vi "Format Error Properties.vi"(8 "error in (no error)":errorcluster, 11 "CtrlTerm Ref":refnum<vi>) -> (0 "error out":errorcluster, 2 "Changed?":bool)   [LabVIEW 2020]
uses:
  <vilib>/Utility/miscctls.llb/LVSelectionTypeDef.ctl
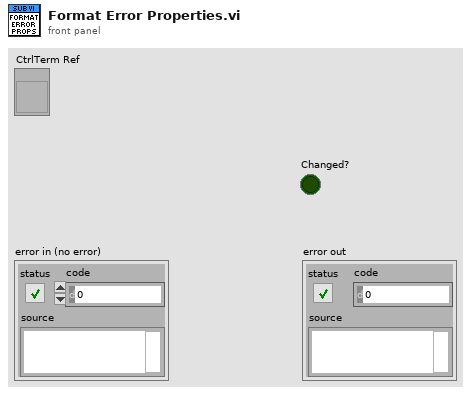
[diagram p1: front panel]
types:
  T1 = typedef "LVSelectionTypeDef.ctl" = cluster{"Selection Start":u32, "Selection End":u32}
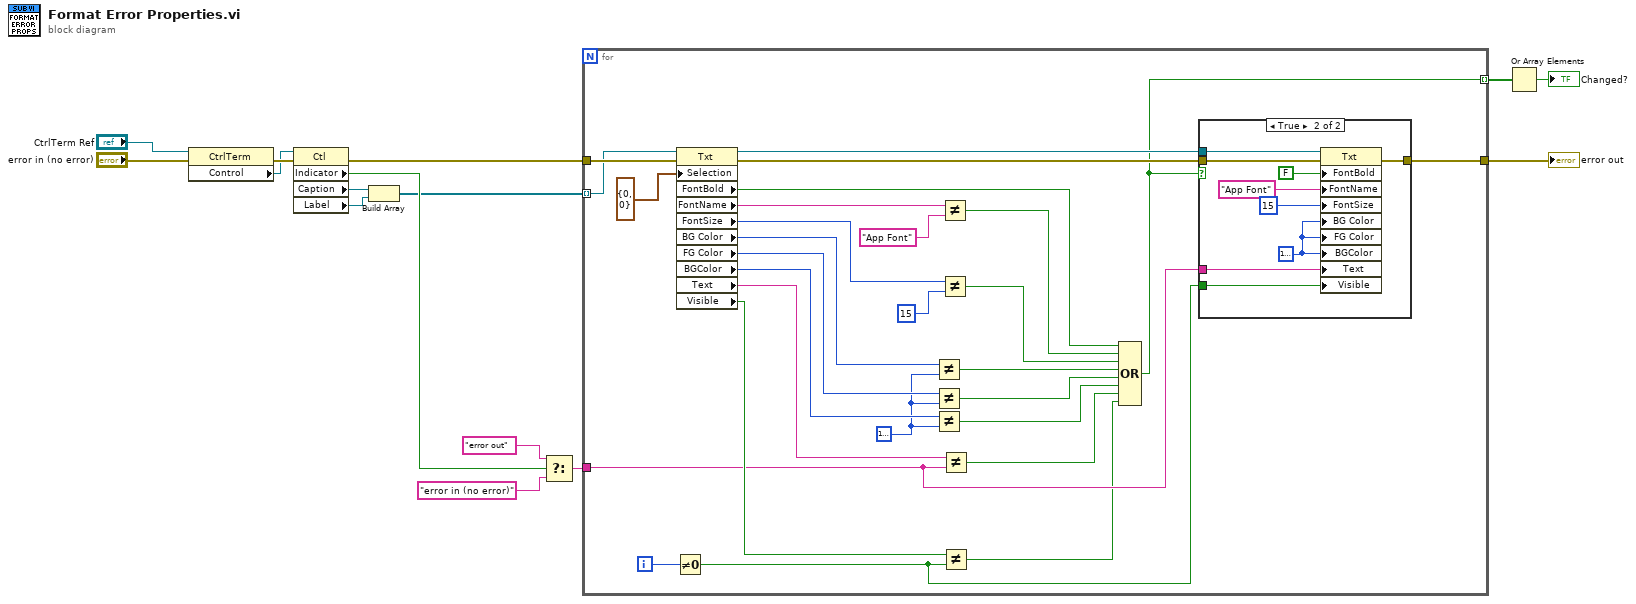
[diagram p0: block diagram]
diagram:
  n1 = property class="CtrlTerm"(reference="CtrlTerm Ref", error in="error in (no error)") -> (error out=w13:errorcluster, "Control"=w12:refnum<vi>)  [unwired: 1 out]
  n2 = property class="Ctl"(reference=w12, error in=w13) -> (error out=w11:errorcluster, "Indicator"=w6:bool, "Caption"=w10:refnum<vi>, "Label"=w9:refnum<vi>)  [unwired: 1 out]
  n3 = Build Array(w10, w9) -> (w5:refnum<vi>[])
  n4 = Select(t="error out", s=w6, f="error in (no error)") -> (s? t:f=w4:string)
  n5 = for {
    tunnel: w11 -> [w26]
    tunnel: w5 -> [w25] mode=indexing
    tunnel: w4 -> [w21]
    tunnel: [w19] -> w3
    tunnel: [w16] -> w2 mode=indexing
    i -> [w24]
    w34 = u32 16777216
    n6 = Not Equal To 0?(x=w24) -> (x != 0?=w20:bool)
    n7 = property class="Txt"(reference=w25, error in=w26, "Selection"=T1 {"Selection Start"=0, "Selection End"=0} ("Label.Selection")) -> (reference out=w43:refnum<vi>, error out=w42:errorcluster, "FontBold"=w37:bool, "FontName"=w32:string, "FontSize"=w30:u32, "BG Color"=w40:u32, "FG Color"=w39:u32, "BGColor"=w35:u32, "Text"=w23:string, "Visible"=w22:bool)
    n8 = Not Equal?(x=w40, y=w34) -> (x != y?=w41:bool)
    n9 = Not Equal?(x=w39, y=w34) -> (x != y?=w38:bool)
    n10 = Not Equal?(x=w35, y=w34) -> (x != y?=w33:bool)
    n11 = Not Equal?(x=w32, y="App Font") -> (x != y?=w27:bool)
    n12 = Not Equal?(x=w30, y=u32 15) -> (x != y?=w28:bool)
    n13 = Not Equal?(x=w23, y=w21) -> (x != y?=w18:bool)
    n14 = Not Equal?(x=w22, y=w20) -> (x != y?=w17:bool)
    n15 = Compound Arithmetic op=OR(w37, w27, w28, w41, w38, w33, w18, w17) -> (w16:bool)
    n16 = case shown="True" w16 {
      tunnel: w43 -> [_ w53]
      tunnel: w42 -> [w44 w52]
      tunnel: [w44 w50] -> w19
      tunnel: w21 -> [_ w46]
      tunnel: w20 -> [_ w45]
      frame False {
      }
      frame True {
        w49 = u32 16777216
        n17 = property class="Txt"(reference=w53, error in=w52, "FontBold"=FALSE ("AutoSize To Fit Contents?"), "FontName"="App Font" ("y"), "FontSize"=u32 15 ("y"), "BG Color"=w49, "FG Color"=w49, "BGColor"=w49, "Text"=w46, "Visible"=w45) -> (error out=w50:errorcluster)  [unwired: 1 out]
      }
    }
  }
  "error out" <- w3
  n18 = Or Array Elements(Boolean array=w2) -> (logical OR=→"Changed?":bool)
